vi "Reset PLL.vi"(7 "index":i32, 8 "error in":errorcluster, 11 "fpga session in":refnum<k20>) -> (0 "error out":errorcluster, 3 "fpga session out":refnum<k20>)   [LabVIEW 2017, in "Lock-In Amplifier Example Host.lvlib"]
uses:
  Lock-In Amplifier Example Host.lvlib
  fpga type.ctl
  <vilib>/Utility/error.llb/Error Cluster From Error Code.vi
  <vilib>/rvi/errors/niLvFpgaAdjustHostInterfaceError.vi
  <vilib>/rvi/interface/nirviReadWriteControl/nirviReadWriteControl.xnode
  NiFpgaLv.dll
  <vilib>/rvi/interface/Simulation/niFpgaSimulationCallBeginRW.vi
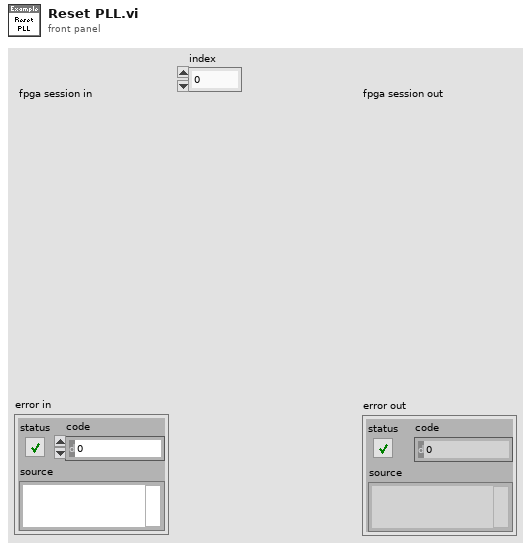
[diagram p1: front panel]
types:
  T1 = typedef "Lock-In Amplifier Example Host.lvlib/fpga type.ctl" = refnum<k20>
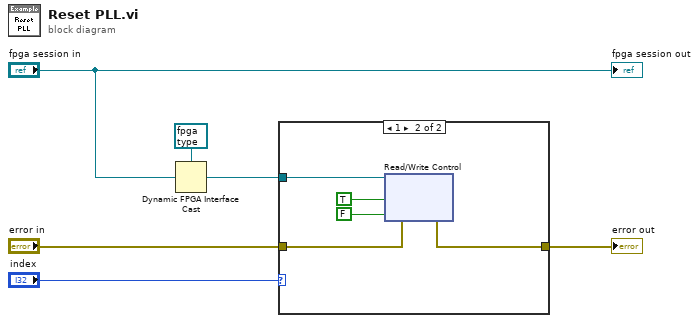
[diagram p0: block diagram]
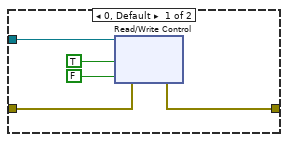
[diagram p2: hidden frame]
diagram:
  n1 = Dynamic FPGA Interface Cast(Session In=T1 refnum ("fpga type"), Type="fpga session in") -> (Session Out=w4:T1)
  n2 = case shown="1" "index" {
    tunnel: w4 -> [w11 w16]
    tunnel: [w10 w15] -> w3
    tunnel: "error in" -> [w8 w13]
    frame 0, Default {
      n3 = xnode "Read/Write Control"("FPGA VI Reference In"=w11, "error in"=w8, "pll.reset 0"=TRUE ("pll.enable 1"), "pll.reset 0"=FALSE) -> ("error out"=w10:errorcluster)  [unwired: 1 out]
    }
    frame 1 {
      n4 = xnode "Read/Write Control"("FPGA VI Reference In"=w16, "error in"=w13, "pll.reset 1"=TRUE ("pll.enable 1"), "pll.reset 1"=FALSE ("pll.reset 0")) -> ("error out"=w15:errorcluster)  [unwired: 1 out]
    }
  }
  "error out" <- w3
  "fpga session out" <- "fpga session in"
